vi "ziTicks2S.vi"   [LabVIEW 2016, in "Zurich Instruments LabOne.lvlib"]
doc: "Convert a scalara or vector value from the machine unit ticks to the SI unit second."
uses:
  Zurich Instruments LabOne.lvlib
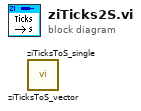
[diagram p0: block diagram]
diagram:
  n1 = call "ziTicksToS_vector.vi"() -> ()  [unwired: 3 in, 3 out]
  n2 = call "ziTicksToS_single.vi"() -> ()  [unwired: 3 in, 3 out]
